vi "Array_Search_For_Num.vi"(0 "N Rows of Data":string[][](array[string])=[["Title1", "Title2"], ["1", "2"]], 5 "Title?":string, 7 "Row(1)":i32=1) -> (4 "index":i32, 8 "number":dbl)   [LabVIEW 2014]
panel:
  out "output array":string[](array[string])
  # "Searches 2D String Array \nLooks for Title in first row\nand converts Data in N(2) row\nto DBL."
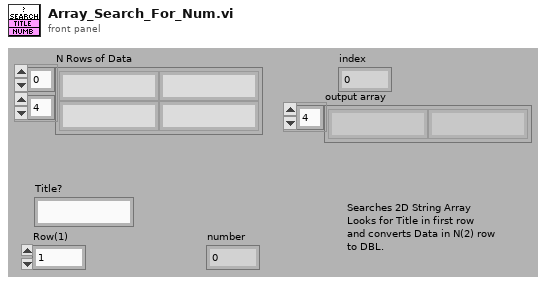
[diagram p1: front panel]
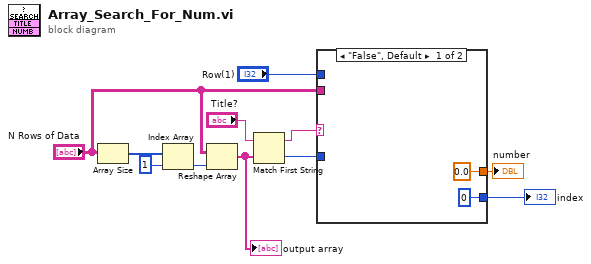
[diagram p0: block diagram]
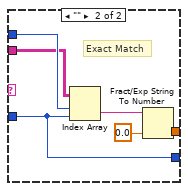
[diagram p2: hidden frame]
diagram:
  n1 = Array Size(array="N Rows of Data") -> (size(s)=w10:i32[])
  n2 = Index Array(array=w10, index=1) -> (element=w8:i32)
  n3 = Reshape Array("N Rows of Data", w8) -> (w6:string[])
  "output array" <- w6
  n4 = Match First String(2:w6, 3:"Title?") -> (0:w4:i32, 1:w2:string)
  n5 = case shown="\"False\", Default" w2 {
    tunnel: "Row(1)" -> [_ w19]
    tunnel: "N Rows of Data" -> [_ w18]
    tunnel: w4 -> [_ w14]
    tunnel: [0.0 w16] -> w3
    tunnel: [0 ("index") w14] -> w1
    frame "False", Default {
    }
    frame "" {
      # "Exact Match"
      n6 = Index Array(array=w18, index (row)=w19, index (col)=w14) -> (element=w17:string)
      n7 = Fract/Exp String To Number(string=w17, default (0 dbl)=0.0 ("default (0 DBL)")) -> (number=w16:dbl)  [unwired: 2 in, 1 out]
    }
  }
  "number" <- w3
  "index" <- w1
